vi "Read UIRef.vi"(8 "error in (no error)":errorcluster, 9 "0Arrive/1Finish":i32, 10 "UI Ref":T1, 11 "LaserDetect01 in":refnum<class "LaserDetect01.lvclass">) -> (0 "error out":errorcluster, 2 "RefOut":refnum<vi>, 3 "LaserDetect01 out":refnum<class "LaserDetect01.lvclass">)   [LabVIEW 2019, in "LaserDetect01.lvclass"]
uses:
  LaserDetect01.lvclass
  Ctrl/Auto Inspection Main UI Ref.ctl
  FlowIOCtrl.lvclass
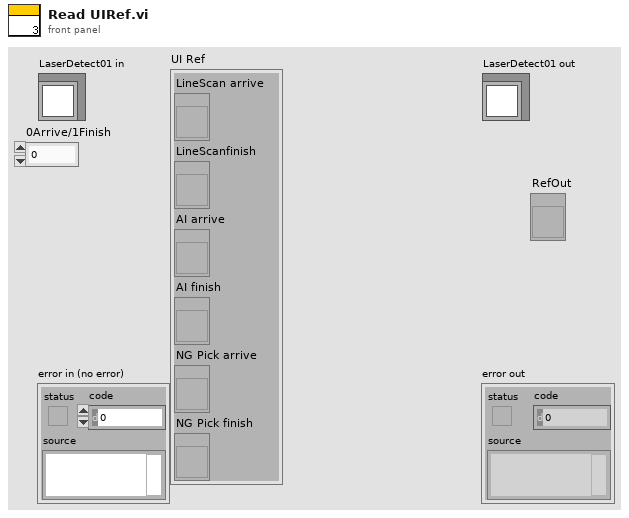
[diagram p1: front panel]
types:
  T1 = typedef "Auto Inspection Main UI Ref.ctl" = cluster{"LineScan arrive":refnum<vi>, "LineScanfinish":refnum<vi>, "AI arrive":refnum<vi>, "AI finish":refnum<vi>, "NG Pick arrive":refnum<vi>, "NG Pick finish":refnum<vi>}
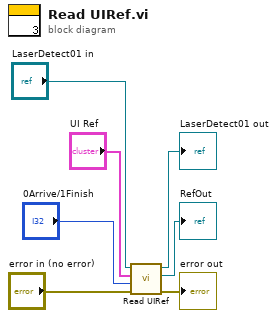
[diagram p0: block diagram]
diagram:
  n1 = call-parent "Read UIRef.vi"("error in (no error)"="error in (no error)", "0Arrive/1Finish"="0Arrive/1Finish", "UI Ref"="UI Ref", "Station Action in"="LaserDetect01 in") -> ("error out"=→"error out":errorcluster, "RefOut"=→"RefOut":refnum<vi>, "Station Action out"=→"LaserDetect01 out":refnum<class "LaserDetect01.lvclass">)  [unwired: 5 in]
